vi "RS.vi"() -> ()   [LabVIEW 2013]
panel:
  out "!Q":bool
  out "Q":bool
  in  "S":bool
  in  "C":bool
  in  "R":bool
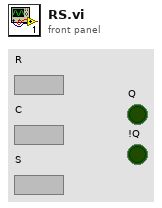
[diagram p1: front panel]
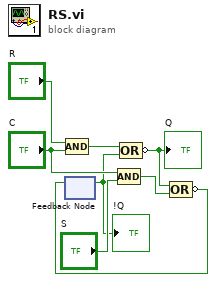
[diagram p0: block diagram]
diagram:
  n1 = feedback #1() -> (w1:bool)  [unwired: 1 in]
  "!Q" <- w1
  n2 = Compound Arithmetic op=AND("R", "C") -> (w5:bool)
  n3 = Compound Arithmetic op=AND("C", "S") -> (w4:bool)
  n4 = Compound Arithmetic op=OR(w5, w1) -> (invert w3:bool)
  "Q" <- w3
  n5 = Compound Arithmetic op=OR(w3, w4) -> (invert w2:bool)
  n6 = feedback-in #1(w2) -> ()
